vi "ElapsedTime.vi"(3 "Reset":bool, 5 "Target time(s)":dbl) -> (0 "Time Elapsed":bool, 2 "Elapsed Time":dbl)   [LabVIEW 2020]
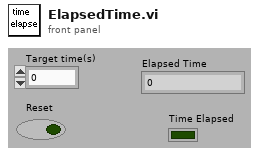
[diagram p1: front panel]
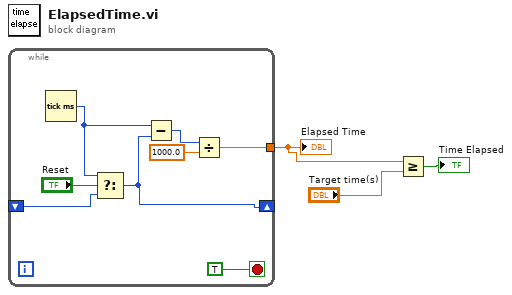
[diagram p0: block diagram]
diagram:
  n1 = while {
    shift-right: [w7] -> _
    shift-left: _ -> [w9]
    tunnel: [w4] -> w3
    stop <- TRUE stop-if-true
    n2 = Tick Count (ms)() -> (millisecond timer value=w8:u32)
    n3 = Select(t=w8, s="Reset", f=w9) -> (s? t:f=w7:u32)
    n4 = Subtract(x=w8, y=w7) -> (x-y=w6:u32)
    n5 = Divide(x=w6, y=1000.0) -> (x/y=w4:dbl)
  }
  "Elapsed Time" <- w3
  n6 = Greater Or Equal?(x=w3, y="Target time(s)") -> (x >= y?=→"Time Elapsed":bool)
